vi "load data3.vi"(7 "Append dataset":bool, 10 "existing file numbers":string[](array[string]), 11 "existing data cluster":cluster{"array type (2D Dbl)":dbl[][]}[](array[cluster])) -> (2 "data names":string[](array[string]), 3 "data cluster":cluster{"all data":dbl[][]}[](array[cluster]))   [LabVIEW 2020]
uses:
  <vilib>/Utility/file.llb/Read Delimited Spreadsheet (DBL).vi
panel:
  out "Start Loading Data files":bool
  in  "Done":bool
  out "# of importe files":i32
  in  "numbered file":T1={"FILE HEADER"="20120217", "FROM"="012", "TO"="012", "Excluding\nFrom"="", "Excluding\nTo"="", "Start Loading Data files"=FALSE}
  in  "Cancel button":bool
  in  "Import Menu":T2(ring)
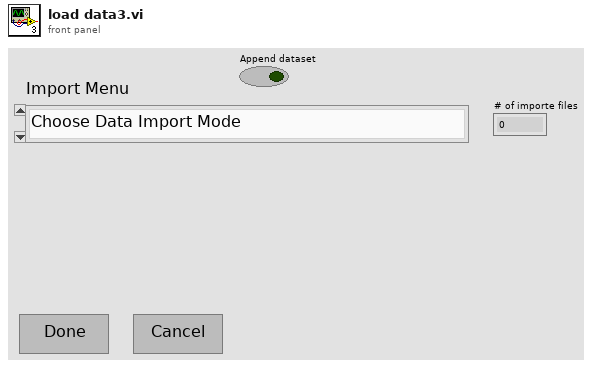
[diagram p1: front panel]
types:
  T1 = cluster{"FILE HEADER":string, "FROM":string, "TO":string, "Excluding\nFrom":string, "Excluding\nTo":string, "Start Loading Data files":bool}
  T2 = enum16{"Choose Data Import Mode", "Numbered NML Data Acq files saved in the drive", "Import current data being taken", "Manual selection of text file(s) ", "Manual Input of single XY plot(s)", "Manual Input of a worksheet"}
  T3 = enum16{"Choose Data Import Mode", "Numbered NML Data Acq files saved in the drive", "Import current NML Data Acq being taken", "Manual selection of text file(s) ", "Manual Input of XY arrays", "Manual Input of a worksheet"}
  T4 = enum16{"Left Button", "Center Button", "Right Button", "Window Close"}
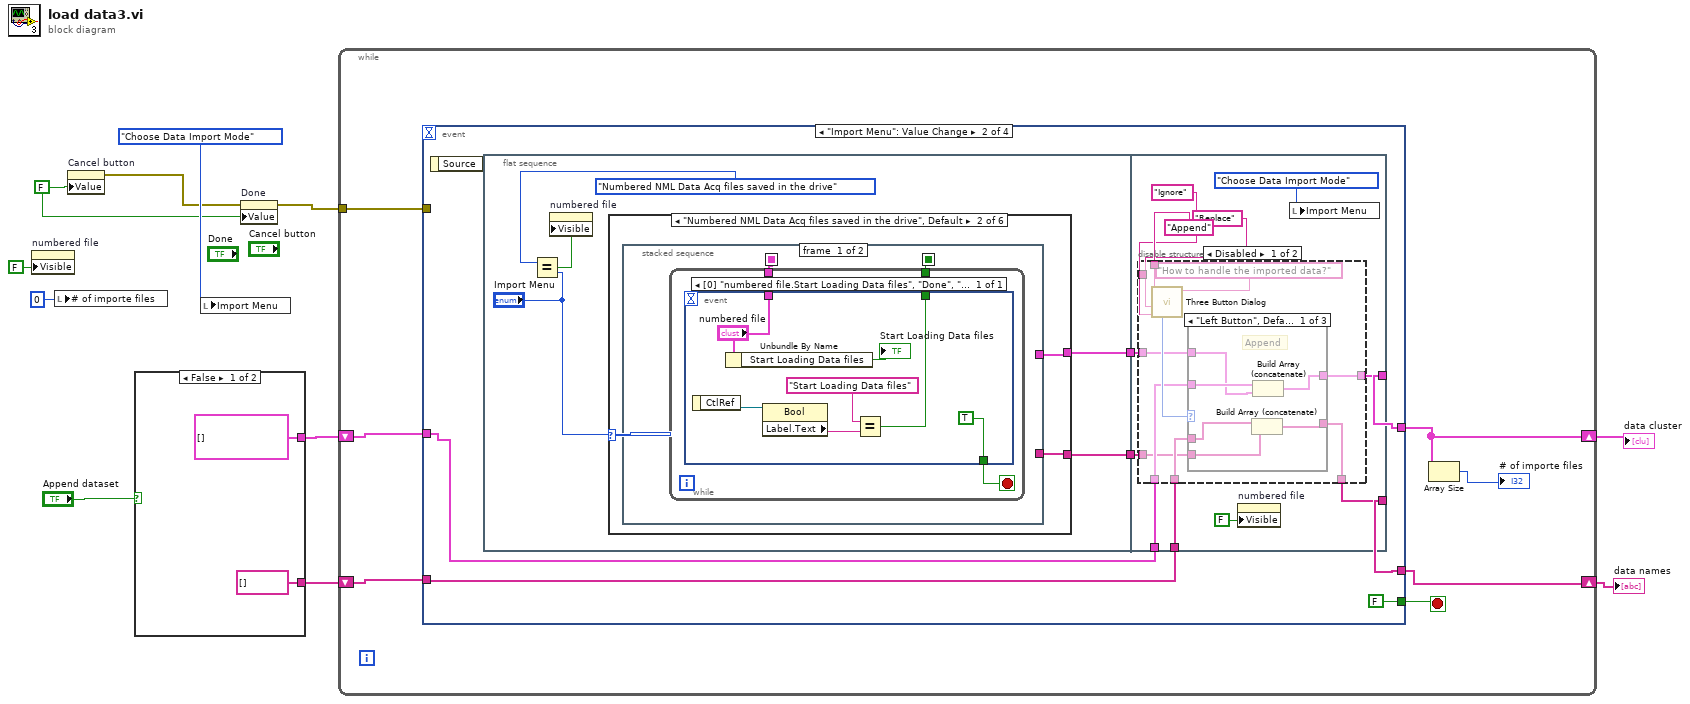
[diagram p0: block diagram]
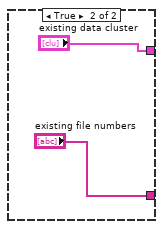
[diagram p2: hidden frame]
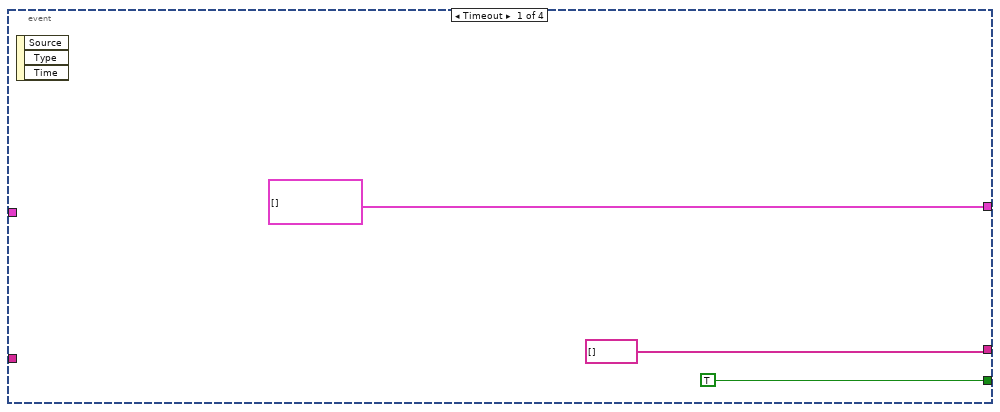
[diagram p3: hidden frame]
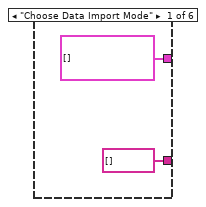
[diagram p4: hidden frame]
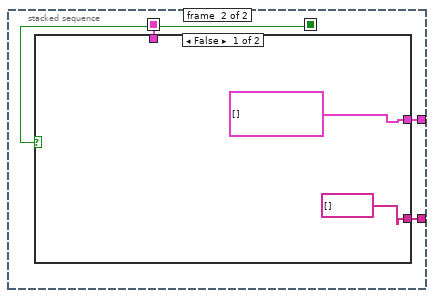
[diagram p5: hidden frame]
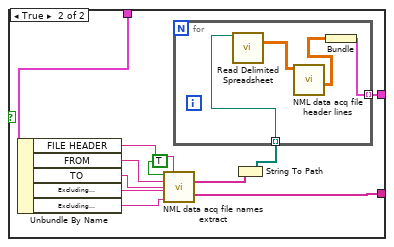
[diagram p6: hidden frame]
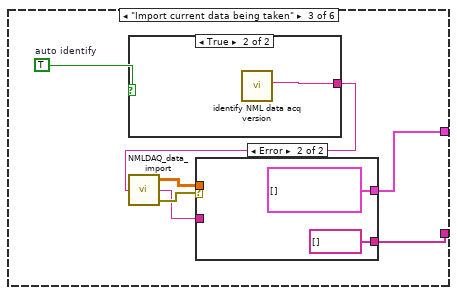
[diagram p7: hidden frame]
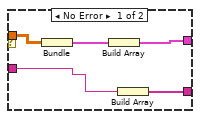
[diagram p8: hidden frame]
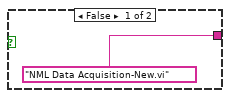
[diagram p9: hidden frame]
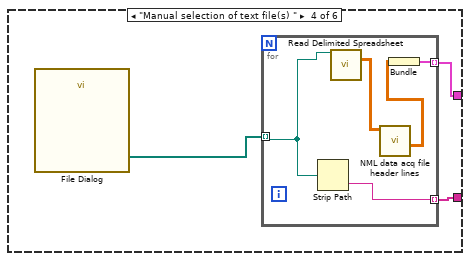
[diagram p10: hidden frame]
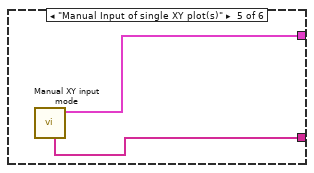
[diagram p11: hidden frame]
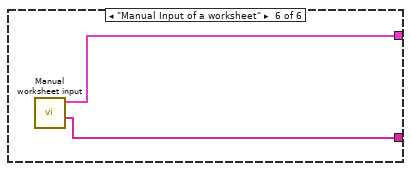
[diagram p12: hidden frame]
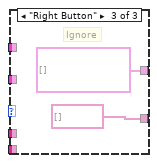
[diagram p14: hidden frame]
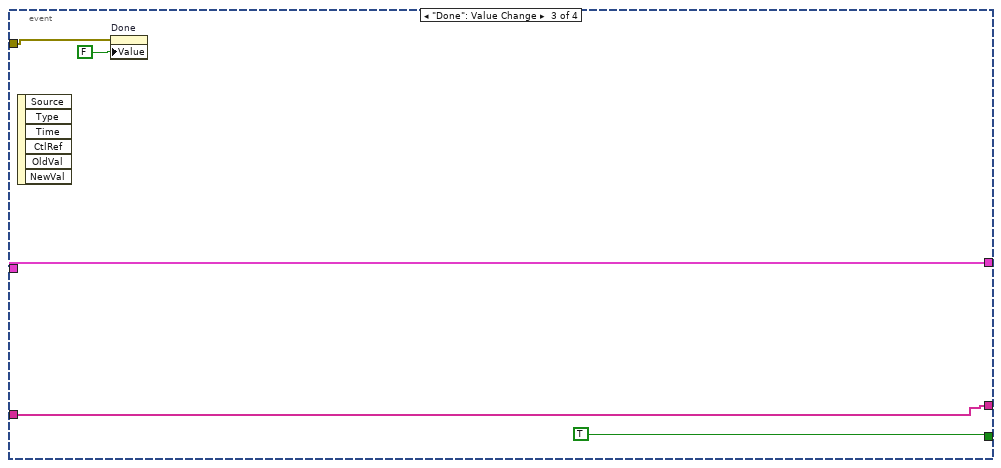
[diagram p16: hidden frame]
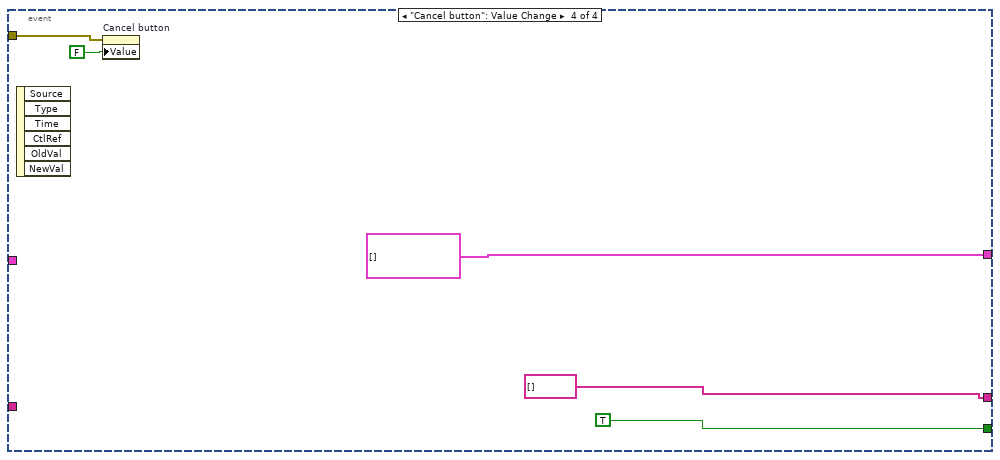
[diagram p17: hidden frame]
diagram:
  w2 = FALSE ("Value (Signaling)")
  n1 = property on="numbered file" class="Clust"("Visible"=FALSE) -> ()  [unwired: 2 in, 2 out]
  n2 = local write "# of importe files"(0 ("# of data files")) -> ()
  n3 = property on="Cancel button" class="Bool (strict)"("Value"=w2) -> (error out=w3:errorcluster)  [unwired: 2 in, 1 out]
  n4 = case shown="False" "Append dataset" {
    tunnel: [cluster{"array type (2D Dbl)":dbl[][]}[] [] ("existing data cluster") "existing data cluster"] -> w6
    tunnel: [string[] [] ("existing file numbers") "existing file numbers"] -> w5
    frame False {
    }
    frame True {
    }
  }
  n5 = local write "Import Menu"(T2."Choose Data Import Mode" ("Import Menu")) -> ()
  n6 = property on="Done" class="Bool (strict)"(error in=w3, "Value"=w2) -> (error out=w1:errorcluster)  [unwired: 1 in, 1 out]
  n7 = while {
    shift-right: [w17] -> w7
    shift-left: w6 -> [w21]
    shift-right: [w18] -> w9
    shift-left: w5 -> [w19]
    tunnel: w1 -> [w16]
    stop <- w22 stop-if-true
    n8 = event shown="[1] \"Import Menu\": Value Change" {
      selector: _ -> [_ _ _ _]
      dyn-events: _ -> [_ _ _ _]
      timeout: _ -> [_ _ _ _]
      tunnel: [TRUE FALSE TRUE TRUE] -> w22
      tunnel: [cluster{"array type (2D Dbl)":dbl[][]}[] [] ("Data clusters") w27 w138 cluster{"array type (2D Dbl)":dbl[][]}[] [] ("Data clusters")] -> w17
      tunnel: w21 -> [_ w29 w138 _]
      tunnel: [string[] [] ("file numbers") w26 w137 string[] [] ("file numbers")] -> w18
      tunnel: w19 -> [_ w28 w137 _]
      tunnel: w16 -> [_ _ w136 w141]
      event Timeout {
        n9 = event-data() -> ()  [unwired: 1 in, 3 out]
      }
      event "Import Menu": Value Change {
        n10 = event-data() -> ()  [unwired: 1 in, 1 out]
        n11 = flat-sequence {
          tunnel: [w35] -> w31
          tunnel: [w34] -> w30
          tunnel: w31 -> [w107]
          tunnel: w30 -> [w108]
          tunnel: w29 -> [w110]
          tunnel: w28 -> [w109]
          tunnel: [w106] -> w27
          tunnel: [w105] -> w26
          frame #0 {
            n12 = Equal?(x=T3."Numbered NML Data Acq files saved in the drive", y="Import Menu") -> (x = y?=w33:bool)
            n13 = property on="numbered file" class="Clust"("Visible"=w33) -> ()  [unwired: 2 in, 2 out]
            n14 = case shown="\"Numbered NML Data Acq files saved in the drive\", Default" "Import Menu" {
              tunnel: [cluster{"array type (2D Dbl)":dbl[][]}[] [] ("Data clusters") w41 w75 w93 w100 w102] -> w35
              tunnel: [string[] [] ("file numbers") w40 w76 w91 w99 w101] -> w34
              frame "Choose Data Import Mode" {
              }
              frame "Numbered NML Data Acq files saved in the drive", Default {
                n15 = stacked-sequence {
                  seq-local: [w43 _] -> [_ w56]
                  seq-local: [w42 _] -> [_ w54]
                  tunnel: [_ w57] -> w41
                  tunnel: [_ w55] -> w40
                  frame #0 {
                    n16 = while {
                      tunnel: [w46] -> w43
                      tunnel: [w44] -> w42
                      stop <- w45 stop-if-true
                      n17 = event shown="[0] \"numbered file.Start Loading Data files\", \"Done\", \"Cancel button\": Value Change" {
                        selector: _ -> [_]
                        dyn-events: _ -> [_]
                        timeout: _ -> [_]
                        tunnel: ["numbered file"] -> w46
                        tunnel: [TRUE] -> w45
                        tunnel: [w47] -> w44
                        event "numbered file.Start Loading Data files", "Done", "Cancel button": Value Change {
                          n18 = event-data() -> ("CtlRef"=w50:refnum<vi>)  [unwired: 1 in]
                          n19 = Unbundle By Name("numbered file") -> ("Start Loading Data files"=→"Start Loading Data files":bool)
                          n20 = property class="Bool"(reference=w50) -> ("Label.Text"=w49:string)  [unwired: 1 in, 2 out]
                          n21 = Equal?(x="Start Loading Data files" ("Label.Text"), y=w49) -> (x = y?=w47:bool)
                        }
                      }
                    }
                  }
                  frame #1 {
                    n22 = case shown="False" w54 {
                      tunnel: [cluster{"array type (2D Dbl)":dbl[][]}[] [] ("Data clusters") w69] -> w57
                      tunnel: w56 -> [_ w66]
                      tunnel: [string[] [] ("file numbers") w60] -> w55
                      frame False {
                      }
                      frame True {
                        n23 = Unbundle By Name(w66) -> ("FILE HEADER"=w65:string, "FROM"=w64:string, "TO"=w63:string, "Excluding\nFrom"=w62:string, "Excluding\nTo"=w61:string)
                        n24 = call "NML data acq file names extract.vi"("assign directory"=TRUE, "File name header"=w65, "From"=w64, "To"=w63, "Excluding From"=w62, "Excluding To"=w61) -> ("file paths"=w67:string[], "existing files"=w60:string[])  [unwired: 6 in, 2 out]
                        n25 = String To Path(string=w67) -> (path=w70:path[])
                        n26 = for {
                          tunnel: w70 -> [w73] mode=indexing
                          tunnel: [w74] -> w69 mode=indexing
                          n27 = call-poly <vilib>:"Read Delimited Spreadsheet.vi"("file path (dialog if empty)"=w73) -> ("all rows"=w72:dbl[][])  [unwired: 9 in, 5 out]
                          n28 = call "NML data acq file header lines.vi"("all rows"=w72) -> ("real data?"=w71:dbl[][])  [unwired: 8 in, 2 out]
                          n29 = Bundle("real data?"=w71) -> (w74:cluster{"real data?":dbl[][]})  [unwired: 1 in]
                        }
                      }
                    }
                  }
                }
              }
              frame "Import current data being taken" {
                w80 = TRUE  # auto identify
                n30 = case shown="True" w80 {
                  tunnel: ["NML Data Acquisition-New.vi" ("NML Data Acquisition VI") w90] -> w81
                  frame False {
                  }
                  frame True {
                    n31 = call "identify NML data acq version.vi"() -> ("NML data in the memory"=w90:string)  [unwired: 11 in]
                  }
                }
                n32 = call "NMLDAQ_data_import.vi"("NML Data Acquisition VI"=w81) -> ("data"=w78:dbl[][], "file name"=w77:string, "error out"=w79:errorcluster)
                n33 = case shown="Error" w79 {
                  tunnel: w78 -> [w85 _]
                  tunnel: w77 -> [w82 _]
                  tunnel: [w84 string[] []] -> w76
                  tunnel: [w83 cluster{"data":dbl[][]}[] []] -> w75
                  frame No Error {
                    n34 = Bundle("data"=w85) -> (w86:cluster{"data":dbl[][]})  [unwired: 1 in]
                    n35 = Build Array(w86) -> (w83:cluster{"data":dbl[][]}[])
                    n36 = Build Array(w82) -> (w84:string[])
                  }
                  frame Error {
                  }
                }
              }
              frame "Manual selection of text file(s) " {
                n37 = call "File Dialog"() -> ("selected paths"=w92:path[])  [unwired: 12 in, 3 out]
                n38 = for {
                  tunnel: w92 -> [w97] mode=indexing
                  tunnel: [w98] -> w93 mode=indexing
                  tunnel: [w96] -> w91 mode=indexing
                  n39 = Strip Path(path=w97) -> (name=w96:string)  [unwired: 1 out]
                  n40 = call-poly <vilib>:"Read Delimited Spreadsheet.vi"("file path (dialog if empty)"=w97) -> ("all rows"=w95:dbl[][])  [unwired: 9 in, 5 out]
                  n41 = call "NML data acq file header lines.vi"("all rows"=w95) -> ("real data?"=w94:dbl[][])  [unwired: 8 in, 2 out]
                  n42 = Bundle("real data?"=w94) -> (w98:cluster{"real data?":dbl[][]})  [unwired: 1 in]
                }
              }
              frame "Manual Input of single XY plot(s)" {
                n43 = call "Manual XY input mode.vi"() -> ("Data clusters"=w100:cluster{"array type (2D Dbl)":dbl[][]}[], "data names"=w99:string[])  [unwired: 7 in, 3 out]
              }
              frame "Manual Input of a worksheet" {
                n44 = call "Manual worksheet input.vi"() -> ("data names"=w101:string[], "Data clusters"=w102:cluster{"array type (2D Dbl)":dbl[][]}[])  [unwired: 8 in, 2 out]
              }
            }
          }
          frame #1 {
            n45 = disable-structure shown="Disabled" {
              disable-tunnel: "Append" ("Left Button Text (\"Yes\")") -> [w123 _]
              disable-tunnel: "Replace" ("Center Button Text (\"No\")") -> [w122 _]
              disable-tunnel: "Ignore" ("Right Button Text (\"Cancel\")") -> [w121 _]
              disable-tunnel: w110 -> [w119 _]
              disable-tunnel: w109 -> [w118 _]
              disable-tunnel: w108 -> [w117 _]
              disable-tunnel: w107 -> [w116 _]
              disable-tunnel: [w115 _] -> w106
              disable-tunnel: [w114 _] -> w105
              frame Disabled {
                n46 = call <vilib>:"Three Button Dialog.vi"("Right Button Text (\"Cancel\")"=w121, "Center Button Text (\"No\")"=w122, "Left Button Text (\"Yes\")"=w123, "message"="How to handle the imported data?") -> ("Which Button?"=w124:T4)  [unwired: 7 in]
                n47 = case shown="\"Left Button\", Default" w124 {
                  tunnel: [w130 w132 cluster{"array type (2D Dbl)":dbl[][]}[] []] -> w115
                  tunnel: [w129 w131 string[] []] -> w114
                  tunnel: w119 -> [w128 _ _]
                  tunnel: w118 -> [w127 _ _]
                  tunnel: w117 -> [w126 w131 _]
                  tunnel: w116 -> [w125 w132 _]
                  frame "Left Button", Default {
                    # "Append"
                    n48 = Build Array (concatenate)(w127, w126) -> (w129:string[])
                    n49 = Build Array (concatenate)(w128, w125) -> (w130:cluster{"array type (2D Dbl)":dbl[][]}[])
                  }
                  frame "Center Button" {
                    # "Replace"
                  }
                  frame "Right Button" {
                    # "Ignore"
                  }
                }
              }
              frame Enabled {
              }
            }
            n50 = property on="numbered file" class="Clust"("Visible"=FALSE) -> ()  [unwired: 2 in, 2 out]
            n51 = local write "Import Menu"(T2."Choose Data Import Mode" ("Import Menu")) -> ()
          }
        }
      }
      event "Done": Value Change {
        n52 = event-data() -> ()  [unwired: 1 in, 6 out]
        n53 = property on="Done" class="Bool (strict)"(error in=w136, "Value"=FALSE ("Value (Signaling)")) -> ()  [unwired: 1 in, 2 out]
      }
      event "Cancel button": Value Change {
        n54 = event-data() -> ()  [unwired: 1 in, 6 out]
        n55 = property on="Cancel button" class="Bool (strict)"(error in=w141, "Value"=FALSE ("Value (Signaling)")) -> ()  [unwired: 1 in, 2 out]
      }
    }
    n56 = Array Size(array=w17) -> (size(s)=→"# of importe files":i32)
  }
  "data cluster" <- w7
  "data names" <- w9
